vi "M01 Wind Turbine.vi"(11 "NXT/EV3":T1) -> (1 "Angle out":sgl=47.0, 3 "EV3 out":T1)   [LabVIEW 2016]
uses:
  <vilib>/NXT/Subs/LVHSConnector.ctl
  <vilib>/NXT/LegoClasses/BrickReference/BrickReference.lvclass
  <vilib>/NXT/Block Support/NXT_OutputPort.ctl
  <vilib>/NXT/Dual Mode Library/Waits/Wait_Num.vi
  <vilib>/NXT/NXTIO Xnodes/AddressXNode/NXTIOAddress.xnode
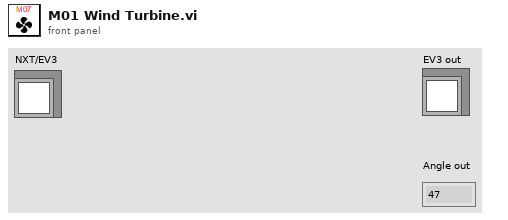
[diagram p1: front panel]
types:
  T1 = typedef "LVHSConnector.ctl" = refnum<class "BrickReference.lvclass">
  T2 = typedef "NXT_OutputPort.ctl" = u8
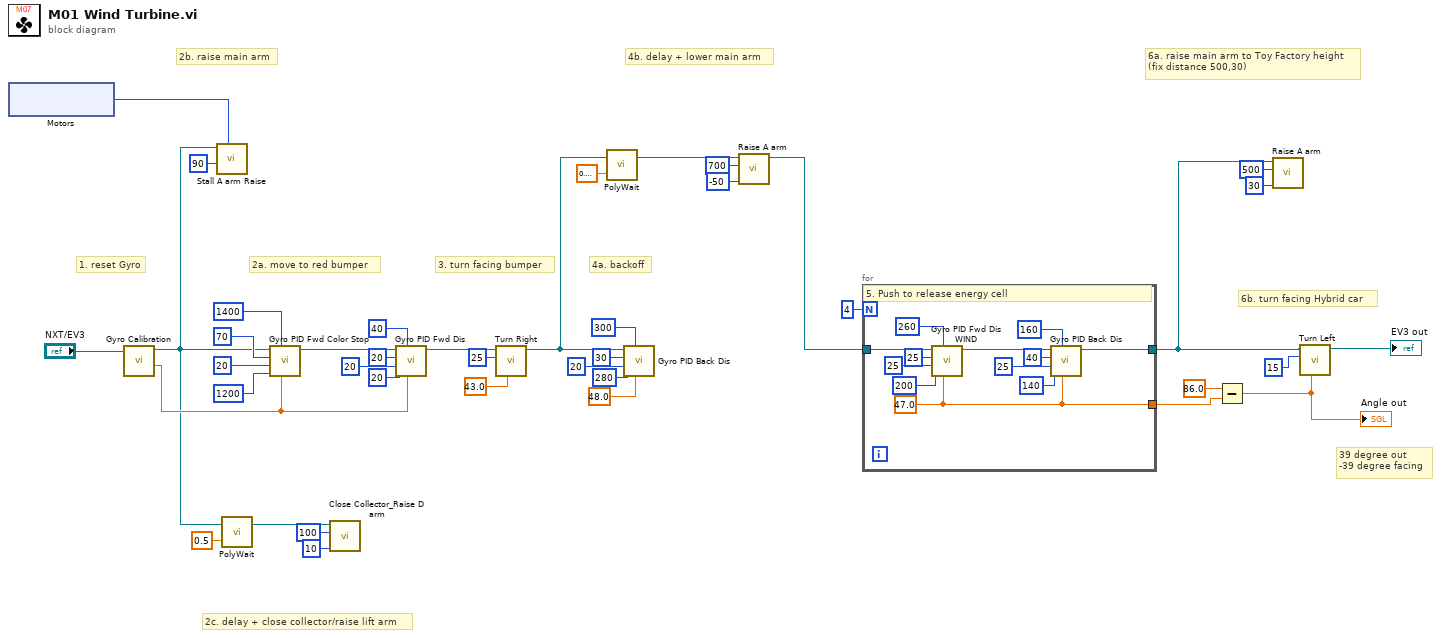
[diagram p0: block diagram]
diagram:
  # "39 degree out\n-39 degree facing"
  # "6b. turn facing Hybrid car"
  # "6a. raise main arm to Toy Factory height\n(fix distance 500,30)"
  # "4b. delay + lower main arm"
  # "4a. backoff"
  # "3. turn facing bumper"
  # "2a. move to red bumper"
  # "2b. raise main arm"
  # "2c. delay + close collector/raise lift arm"
  # "1. reset Gyro"
  n1 = xnode "Motors"() -> ("Motor"=w12:T2)
  n2 = call "Gyro Calibration.vi"("NXT/EV3"="NXT/EV3") -> ("Degrees"=w34:sgl, "NXT/EV3"=w17:T1)  [unwired: 6 in, 1 out]
  n3 = call "Stall A arm Raise.vi"("Port (Port A)"=w12, "Power"=i8 90, "NXT/EV3"=w17) -> ()  [unwired: 8 in, 1 out]
  n4 = call-poly <vilib>:"PolyWait.vi"("Time (1 sec)"=sgl 0.5, "NXT/EV3"=w17) -> ("NXT/EV3"=w10:T1)  [unwired: 2 in]
  n5 = call "Gyro PID Fwd Color Stop.vi"("Target angle"=w34, "Threshold to Color"=1400 ("Threshold to C1"), "Threshold to slow"=1200 ("Threshold to De-acc"), "Min. speed"=20 ("De-acc"), "Max. speed"=70 ("Acc"), "EV3 in"=w17) -> ("EV3 out"=w38:T1)  [unwired: 5 in]
  n6 = call "Close Collector_Raise D arm.vi"("Power"=i8 10, "Rotation"=100, "EV3 in"=w10) -> ()  [unwired: 8 in, 1 out]
  n7 = call "Gyro PID Fwd Dis.vi"("Target angle"=w34, "Threshold to stop"=40 ("Stop rotation"), "Threshold to slow"=20 ("Threshold to De-acc"), "Min. speed"=20 ("De-acc"), "Max. speed"=20 ("Acc"), "EV3 in"=w38) -> ("EV3 out"=w33:T1)  [unwired: 5 in]
  n8 = call "Turn Right.vi"("Turning angle"=sgl 43.0, "Motor B (right)"=i8 25, "EV3 in"=w33) -> ("EV3 out"=w11:T1)  [unwired: 8 in]
  n9 = call-poly <vilib>:"PolyWait.vi"("Time (1 sec)"=sgl 0.6, "NXT/EV3"=w11) -> ("NXT/EV3"=w7:T1)  [unwired: 2 in]
  n10 = call "Gyro PID Back Dis.vi"("Target angle"=sgl 48.0 ("Ini. Degrees"), "Threshold to stop"=300 ("Stop rotation"), "Threshold to slow"=280 ("Threshold to De-acc"), "Min. speed"=20 ("De-acc"), "Max. speed"=30 ("Acc"), "EV3 in"=w11) -> ()  [unwired: 5 in, 1 out]
  n11 = call "Raise A arm.vi"("Power"=i8 -50, "Rotation"=700, "EV3 in"=w7) -> ("EV3 out"=w4:T1)  [unwired: 8 in]
  n12 = for {
    N: 4 -> [_]
    tunnel: [w45] -> w1
    tunnel: [w44] -> w23
    tunnel: w4 -> [w42]
    w44 = sgl 47.0 ("Ini. Degrees")
    # "5. Push to release energy cell"
    n13 = call "Gyro PID Fwd Dis WIND.vi"("Target angle"=w44, "Threshold to stop"=260 ("Stop rotation"), "Threshold to slow"=200 ("Threshold to De-acc"), "Higher speed"=25 ("De-acc"), "Max. speed"=25 ("Acc"), "EV3 in"=w42) -> ("EV3 out"=w46:T1)  [unwired: 5 in]
    n14 = call "Gyro PID Back Dis.vi"("Target angle"=w44, "Threshold to stop"=160 ("Stop rotation"), "Threshold to slow"=140 ("Threshold to De-acc"), "Min. speed"=25 ("De-acc"), "Max. speed"=40 ("Acc"), "EV3 in"=w46) -> ("EV3 out"=w45:T1)  [unwired: 5 in]
  }
  n15 = Subtract(x=86.0, y=w23) -> (x-y=w21:dbl)
  "Angle out" <- w21
  n16 = call "Raise A arm.vi"("Power"=i8 30, "Rotation"=500, "EV3 in"=w1) -> ()  [unwired: 8 in, 1 out]
  n17 = call "Turn Left.vi"("Turning angle"=w21, "Motor B (right)"=i8 15, "EV3 in"=w1) -> ("EV3 out"=→"EV3 out":T1)  [unwired: 8 in]
